vi "SS2 Live_Download Single Image.vi"(4 "# 8-bit Images (1)":i32=1, 6 "Block Size":i32=-1, 8 "Error In":errorcluster, 9 "Discard First Image":bool=TRUE, 10 "Image":T1, 11 "Device Refnum":refnum<k24>) -> (0 "Error Out":errorcluster, 2 "Image Out":T1)   [LabVIEW 2019]
uses:
  C:/UCLA Thinkpad Google Drive/LabVIEW 2019 SP1/builds/SS2 Live Distribution/Opal Kelly/C# Wrapper/libFrontPanel-csharp.dll
  Opal Kelly/C# Wrapper/libFrontPanel-csharp.dll
  <vilib>/vision/Image Controls.llb/IMAQ Image.ctl
  8f499a87-0ce6-40db-98f3-8f764b7e409e.vi
  <vilib>/Utility/High Resolution Relative Seconds.vi
  Opal Kelly/C# Wrapper/okFrontPanelC#Wrapper.lvlib
panel:
  out "CPU/Image":dbl
  out "ReadFromBlockPipeOut":i32
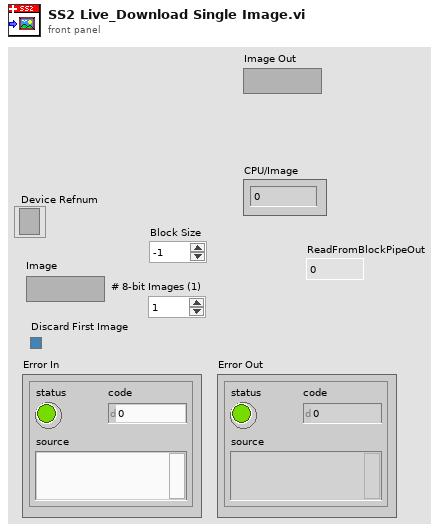
[diagram p1: front panel]
types:
  T1 = typedef "IMAQ Image.ctl" = refnum<image>
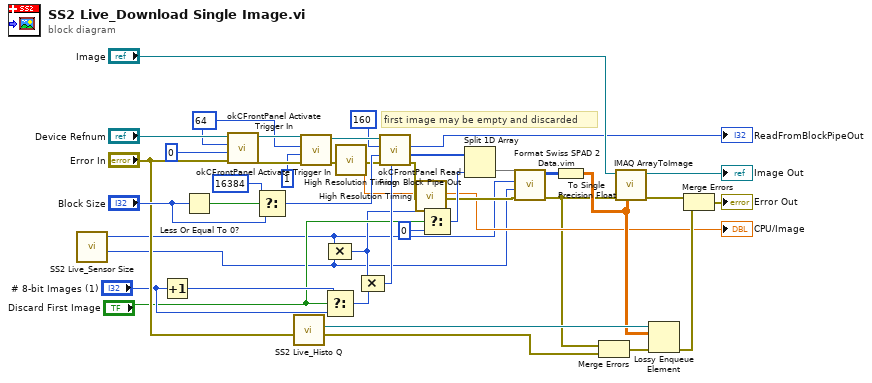
[diagram p0: block diagram]
diagram:
  w40 = 64 ("Endpoint Addr")
  # "first image may be empty and discarded"
  n1 = call "SS2 Live_Sensor Size.vi"() -> ("Y size"=w2:i32, "X size"=w1:i32)  [unwired: 10 in]
  n2 = Increment(x="# 8-bit Images (1)") -> (x+1=w17:i32)
  n3 = Less Or Equal To 0?(x="Block Size") -> (x <= 0?=w31:bool)
  n4 = call "okCFrontPanel Activate Trigger In.vi"("Error In"="Error In", "Bit"=0, "Endpoint Addr"=w40, "okCFrontPanel Refnum"="Device Refnum") -> ("Error Out"=w42:errorcluster, "okCFrontPanel Refnum"=w41:refnum<k24>)  [unwired: 6 in]
  n5 = Select(t=16384, s=w31, f="Block Size") -> (s? t:f=w30:i32)
  n6 = call "SS2 Live_Histo Q.vi"("error in (no error)"="Error In") -> ("error out"=w20:errorcluster, "SS2 Live Histo Q"=w26:refnum<queue>)  [unwired: 5 in]
  n7 = call "okCFrontPanel Activate Trigger In.vi"("Error In"=w42, "Bit"=1, "Endpoint Addr"=w40, "okCFrontPanel Refnum"=w41) -> ("Error Out"=w11:errorcluster, "okCFrontPanel Refnum"=w37:refnum<k24>)  [unwired: 6 in]
  n8 = Select(t=w17, s="Discard First Image", f="# 8-bit Images (1)") -> (s? t:f=w16:i32)
  n9 = Compound Arithmetic op=MULTIPLY(w1, w2) -> (w14:i32)
  n10 = call "High Resolution Timing.vi"("Error In"=w11) -> ("elapsed (relative) seconds"=w7:dbl, "Error Out"=w10:errorcluster)  [unwired: 16 in, 1 out]
  n11 = Compound Arithmetic op=MULTIPLY(w14, w16) -> (w27:i32)
  n12 = call "okCFrontPanel Read From Block Pipe Out.vi"("Length"=w27, "Error In"=w10, "Block Size"=w30, "Endpoint Addr"=160, "okCFrontPanel Refnum"=w37) -> ("Error Out"=w9:errorcluster, "BYTEARRAY"=w34:u8[], "ReadFromBlockPipeOut"=→"ReadFromBlockPipeOut":i32)  [unwired: 3 in, 1 out]
  n13 = call "High Resolution Timing.vi"("relative seconds (NaN)"=w7, "Error In"=w9) -> ("elapsed (relative) seconds"=→"CPU/Image":dbl, "Error Out"=w8:errorcluster)  [unwired: 15 in, 1 out]
  n14 = Select(t=w14, s="Discard First Image", f=0) -> (s? t:f=w12:i32)
  n15 = Split 1D Array(array=w34, index=w12) -> (second subarray=w28:u8[])  [unwired: 1 out]
  n16 = call "Format Swiss SPAD 2 Data.vim"("Error In"=w8, "Y Resolution"=w2, "X Resolution"=w1, "Flattened Image"=w28) -> ("Error Out"=w5:errorcluster, "Image out"=w4:u8[][])  [unwired: 6 in]
  n17 = To Single Precision Float(number=w4) -> (single precision float=w25:sgl[][])
  n18 = Merge Errors(w5, w20) -> (w21:errorcluster)
  n19 = call "IMAQ ArrayToImage"("Image Pixels (Float)"=w25, "error in (no error)"=w5, "Image"="Image") -> ("error out"=w32:errorcluster, "Image Out"=→"Image Out":T1)  [unwired: 7 in]
  n20 = Lossy Enqueue Element(queue=w26, element=w25, error in (no error)=w21) -> (error out=w23:errorcluster)  [unwired: 3 out]
  n21 = Merge Errors(w32, w23) -> (→"Error Out":errorcluster)
